vi "Untitled 1.vi"() -> ()   [LabVIEW 2013]
uses:
  classes/baseClass/propertyDef.ctl
  classes/baseClass/types.ctl
  classes/CS/CS.lvclass
  classes/GenLVOOP/GenLVOOP.lvclass
  classes/baseClass/baseClass.lvclass
  classes/baseParser/baseParser.lvclass
  classes/ProjectHandler.lvlib
panel:
  out "Accessors:Properties":T1[][](array[typedef])
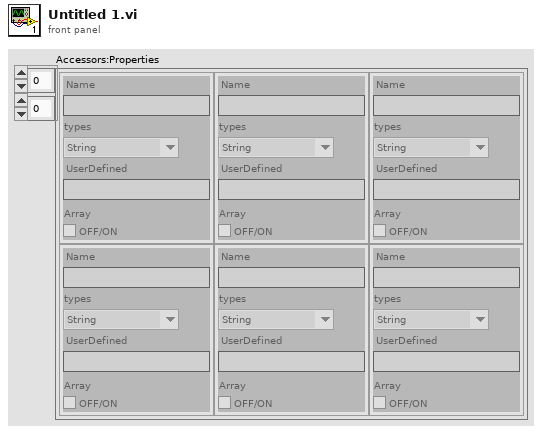
[diagram p1: front panel]
types:
  T1 = typedef "baseClass.lvclass/propertyDef.ctl" = cluster{"Name":string, "types":T2, "UserDefined":string, "Array":bool}
  T2 = typedef "baseClass.lvclass/types.ctl" = enum16{"String", "Int32", "Uint32", "Array", "Class", "Double", "Enum"}
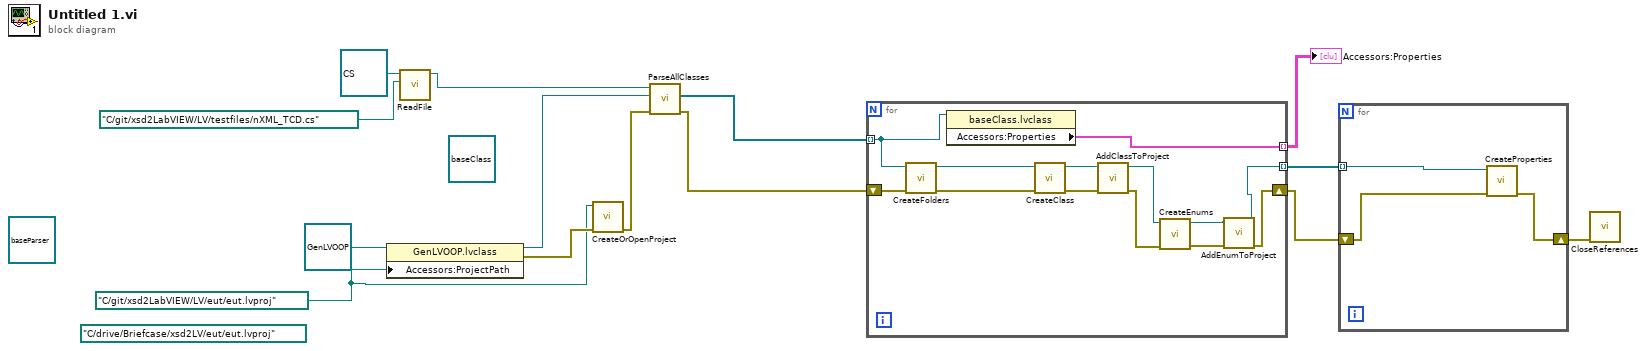
[diagram p0: block diagram]
diagram:
  (unwired) path "C:/drive/Briefcase/xsd2LV/eut/eut.lvproj" ("ProjectPath")
  w1 = path "C:/git/xsd2LabVIEW/LV/eut/eut.lvproj" ("ProjectPath")
  (unwired) refnum<class "baseParser.lvclass"> refnum ("baseParser in")
  (unwired) refnum<class "baseClass.lvclass"> refnum ("cClass in")
  n1 = property class="GenLVOOP.lvclass"(reference=refnum<class "GenLVOOP.lvclass"> refnum ("GenLVOOP.lvclass"), "Accessors:ProjectPath"=w1) -> (reference out=w11:refnum<class "GenLVOOP.lvclass">, error out=w9:errorcluster)  [unwired: 1 in]
  n2 = call-dynamic "ReadFile.vi"("file"=path "C:/git/xsd2LabVIEW/LV/testfiles/nXML_TCD.cs", "baseParser in"=refnum<class "CS.lvclass"> refnum ("CS.lvclass")) -> ("baseParser out"=w12:refnum<class "CS.lvclass">)  [unwired: 8 in, 1 out]
  n3 = call "CreateOrOpenProject.vi"("error in (no error)"=w9, "ProjectPath"=w1) -> ("error out"=w8:errorcluster)  [unwired: 9 in]
  n4 = call-dynamic "ParseAllClasses.vi"("error in (no error)"=w8, "baseClass"=w11, "CS in"=w12) -> ("error out"=w7:errorcluster, "AllClasses"=w10:refnum<class "baseClass.lvclass">[])  [unwired: 6 in, 1 out]
  n5 = for {
    tunnel: w10 -> [w22] mode=indexing
    shift-right: [w17] -> w5
    shift-left: w7 -> [w27]
    tunnel: [w21] -> w6 mode=indexing
    tunnel: [w15] -> w3 mode=indexing
    n6 = call "CreateFolders.vi"("error in (no error)"=w27, "baseClass in"=w22) -> ("error out"=w25:errorcluster, "baseClass out"=w26:refnum<class "baseClass.lvclass">)  [unwired: 8 in]
    n7 = property class="baseClass.lvclass"(reference=w22) -> ("Accessors:Properties"=w21:T1[])  [unwired: 1 in, 2 out]
    n8 = call-dynamic "CreateClass.vi"("error in (no error)"=w25, "baseClass in"=w26) -> ("error out"=w24:errorcluster, "baseClass out"=w23:refnum<class "baseClass.lvclass">)  [unwired: 8 in]
    n9 = call-dynamic "AddClassToProject.vi"("error in (no error)"=w24, "baseClass in"=w23) -> ("error out"=w19:errorcluster, "baseClass out"=w20:refnum<class "baseClass.lvclass">)  [unwired: 8 in]
    n10 = call-dynamic "CreateEnums.vi"("error in (no error)"=w19, "baseClass in"=w20) -> ("error out"=w18:errorcluster, "baseClass out"=w16:refnum<class "baseClass.lvclass">)  [unwired: 8 in]
    n11 = call-dynamic "AddEnumToProject.vi"("error in (no error)"=w18, "baseClass in"=w16) -> ("error out"=w17:errorcluster, "baseClass out"=w15:refnum<class "baseClass.lvclass">)  [unwired: 8 in]
  }
  "Accessors:Properties" <- w6
  n12 = for {
    shift-right: [w29] -> w4
    shift-left: w5 -> [w28]
    tunnel: w3 -> [w30] mode=indexing
    n13 = call-dynamic "CreateProperties.vi"("error in (no error)"=w28, "baseClass in"=w30) -> ("error out"=w29:errorcluster)  [unwired: 8 in, 1 out]
  }
  n14 = call "CloseReferences.vi"("error in (no error)"=w4) -> ()  [unwired: 10 in, 1 out]
